vi "Set Sciscan Scope Image Equalization.vi"(5 "Red Channel":cluster{dbl, dbl}(slide)={0.0, 7.070707070707071} caption="Red Channel Equalizer" scale=-32768.0..32767.0, 7 "Green Channel":cluster{dbl, dbl}(slide)={0.0, 7.070707070707071} caption="Green Channel Equalizer" scale=-32768.0..32767.0, 8 "error in":errorcluster, 9 "Auto Adjust Red":bool, 10 "Auto Adjust Green":bool, 11 "GFG Refnum":refnum<vi>) -> (0 "error out":errorcluster, 3 "GFG Refnum Out":refnum<vi>)   [LabVIEW 2012, in "Sciscan Scope Daemon.lvlib"]
uses:
  Sciscan Scope Daemon.lvlib
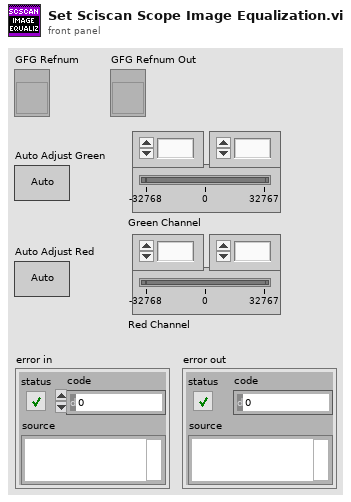
[diagram p1: front panel]
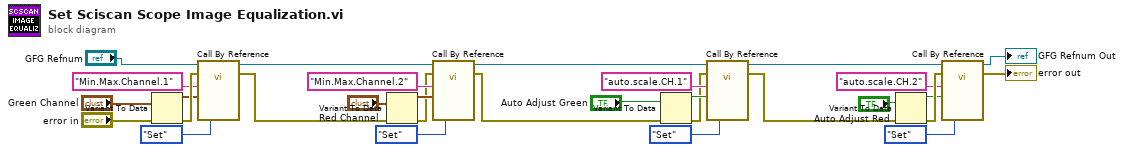
[diagram p0: block diagram]
diagram:
  n1 = Variant To Data(error in="error in", type="Green Channel", Variant="Green Channel") -> (data=w29:cluster{dbl, dbl}, error out=w30:errorcluster)
  n2 = call-by-ref "?"(reference="GFG Refnum", error in=w30, "Variable Name in"="Min.Max.Channel.1", "Variant in"=w29, "Action"=enum16{"Init", "Set", "Get"}."Set") -> (reference out=w17:refnum<vi>, error out=w19:errorcluster)  [unwired: 10 in, 7 out]
  n3 = Variant To Data(error in=w19, type="Red Channel", Variant="Red Channel") -> (data=w21:cluster{dbl, dbl}, error out=w20:errorcluster)
  n4 = call-by-ref "?"(reference=w17, error in=w20, "Variable Name in"="Min.Max.Channel.2", "Variant in"=w21, "Action"=enum16{"Init", "Set", "Get"}."Set") -> (reference out=w4:refnum<vi>, error out=w5:errorcluster)  [unwired: 10 in, 7 out]
  n5 = Variant To Data(error in=w5, type="Auto Adjust Green", Variant="Auto Adjust Green") -> (data=w9:bool, error out=w8:errorcluster)
  n6 = call-by-ref "?"(reference=w4, error in=w8, "Variable Name in"="auto.scale.CH.1", "Variant in"=w9, "Action"=enum16{"Init", "Set", "Get"}."Set") -> (reference out=w3:refnum<vi>, error out=w16:errorcluster)  [unwired: 10 in, 7 out]
  n7 = Variant To Data(error in=w16, type="Auto Adjust Red", Variant="Auto Adjust Red") -> (data=w14:bool, error out=w15:errorcluster)
  n8 = call-by-ref "?"(reference=w3, error in=w15, "Variable Name in"="auto.scale.CH.2", "Variant in"=w14, "Action"=enum16{"Init", "Set", "Get"}."Set") -> (reference out=→"GFG Refnum Out":refnum<vi>, error out=→"error out":errorcluster)  [unwired: 10 in, 7 out]
